vi "update_kineticslength_exp.vi"(1 "NewVal":dbl, 2 "cluster in":T1={"Kinetics"=[], "Spectrum"=[], "Experiments groups"=[], "GRAPH EXPERIMENTAL DATA"=[], "error out"={"status"=FALSE, "code"=0, "source"=""}, "group"=0, "exp selected"=0, "# exp"=0, "kinetics plot names"=[], "spectra plot names"=[], "FromToWave"={"FromWave"=0.0, "ToWave"=0.0}, "GRAPH EXPERIMENTAL DATA ref"=refnum, "timedelays"=[0.0, 0.0, 0.0, 0.0, 0.0, 0.0, 0.0, 0.06019061100911815, 0.0521779104562645, 0.045231877429679615, 0.03921051490799832, 0.033990728811568754, 0.029465811603150715, 0.025543260876973825, 0.02214288834180205, 0.01919518054014414, 0.016639877791965713, 0.014424742312398925, 0.012504490320209958, 0.010839866306230088, 0.009396840537117498, 0.008145913389103785, 0.00706151229029317, 0.006121468943269439, 0.005306566140927374, 0.004600144911132549, 0.003987763959109073, 0.0034569044455719407, 0.00299671406541447, 0.0025977851951783253, 0.0022519625739982996, 0.00195217658646366, 0.0016922987392150965, 0.0014670163768006634, 0.0012717240756200802, 0.0011024294957352762, 0.0009556717658856477, 0.0008284507332614981, 0.0007181656316962257, 0.0006225619144775864, 0.0005396851648867825, 0.00046784114226338394, 0.0004055611468220084, 0.0003515719951773376, 0.00030476999279031153, 0.00026419837125694315, 0.00022902772919263772, 0.0001985390768670671, 0.0001721091379728629, 0.00014919760805372974, 0.00012933610911736794], "wavelengths"=[0.0, 0.0, 0.0, 0.0, 0.0, 0.0, 0.0, 0.06019061100911815, 0.0521779104562645, 0.045231877429679615, 0.03921051490799832, 0.033990728811568754, 0.029465811603150715, 0.025543260876973825, 0.02214288834180205, 0.01919518054014414, 0.016639877791965713, 0.014424742312398925, 0.012504490320209958, 0.010839866306230088, 0.009396840537117498, 0.008145913389103785, 0.00706151229029317, 0.006121468943269439, 0.005306566140927374, 0.004600144911132549, 0.003987763959109073, 0.0034569044455719407, 0.00299671406541447, 0.0025977851951783253, 0.0022519625739982996, 0.00195217658646366, 0.0016922987392150965, 0.0014670163768006634, 0.0012717240756200802, 0.0011024294957352762, 0.0009556717658856477, 0.0008284507332614981, 0.0007181656316962257, 0.0006225619144775864, 0.0005396851648867825, 0.00046784114226338394, 0.0004055611468220084, 0.0003515719951773376, 0.00030476999279031153, 0.00026419837125694315, 0.00022902772919263772, 0.0001985390768670671, 0.0001721091379728629, 0.00014919760805372974, 0.00012933610911736794], "Experiment"=refnum, "Commentaires exp"=refnum, "FromToDelay"={"FromDelay"=0.0, "ToDelay"=0.0}, "cluster tasks DAQmx"={"Heater alaram task"="", "Laser shutter task"="", "Motor task"="", "Accelerator shutter task"="", "Relay key task"="", "Faraday cup task"=""}}) -> (0 "cluster out":T1={"Kinetics"=[], "Spectrum"=[], "Experiments groups"=[], "GRAPH EXPERIMENTAL DATA"=[], "error out"={"status"=FALSE, "code"=0, "source"=""}, "group"=0, "exp selected"=0, "# exp"=0, "kinetics plot names"=[], "spectra plot names"=[], "FromToWave"={"FromWave"=0.0, "ToWave"=0.0}, "GRAPH EXPERIMENTAL DATA ref"=refnum, "timedelays"=[0.0, 0.0, 0.0, 0.0, 0.0, 0.0, 0.0, 0.06019061100911815, 0.0521779104562645, 0.045231877429679615, 0.03921051490799832, 0.033990728811568754, 0.029465811603150715, 0.025543260876973825, 0.02214288834180205, 0.01919518054014414, 0.016639877791965713, 0.014424742312398925, 0.012504490320209958, 0.010839866306230088, 0.009396840537117498, 0.008145913389103785, 0.00706151229029317, 0.006121468943269439, 0.005306566140927374, 0.004600144911132549, 0.003987763959109073, 0.0034569044455719407, 0.00299671406541447, 0.0025977851951783253, 0.0022519625739982996, 0.00195217658646366, 0.0016922987392150965, 0.0014670163768006634, 0.0012717240756200802, 0.0011024294957352762, 0.0009556717658856477, 0.0008284507332614981, 0.0007181656316962257, 0.0006225619144775864, 0.0005396851648867825, 0.00046784114226338394, 0.0004055611468220084, 0.0003515719951773376, 0.00030476999279031153, 0.00026419837125694315, 0.00022902772919263772, 0.0001985390768670671, 0.0001721091379728629, 0.00014919760805372974, 0.00012933610911736794], "wavelengths"=[0.0, 0.0, 0.0, 0.0, 0.0, 0.0, 0.0, 0.06019061100911815, 0.0521779104562645, 0.045231877429679615, 0.03921051490799832, 0.033990728811568754, 0.029465811603150715, 0.025543260876973825, 0.02214288834180205, 0.01919518054014414, 0.016639877791965713, 0.014424742312398925, 0.012504490320209958, 0.010839866306230088, 0.009396840537117498, 0.008145913389103785, 0.00706151229029317, 0.006121468943269439, 0.005306566140927374, 0.004600144911132549, 0.003987763959109073, 0.0034569044455719407, 0.00299671406541447, 0.0025977851951783253, 0.0022519625739982996, 0.00195217658646366, 0.0016922987392150965, 0.0014670163768006634, 0.0012717240756200802, 0.0011024294957352762, 0.0009556717658856477, 0.0008284507332614981, 0.0007181656316962257, 0.0006225619144775864, 0.0005396851648867825, 0.00046784114226338394, 0.0004055611468220084, 0.0003515719951773376, 0.00030476999279031153, 0.00026419837125694315, 0.00022902772919263772, 0.0001985390768670671, 0.0001721091379728629, 0.00014919760805372974, 0.00012933610911736794], "Experiment"=refnum, "Commentaires exp"=refnum, "FromToDelay"={"FromDelay"=0.0, "ToDelay"=0.0}, "cluster tasks DAQmx"={"Heater alaram task"="", "Laser shutter task"="", "Motor task"="", "Accelerator shutter task"="", "Relay key task"="", "Faraday cup task"=""}})   [LabVIEW 2015]
uses:
  Classes/Experiment.lvclass
  Classes/Experiments_group.lvclass
  controls/control-cluster.ctl
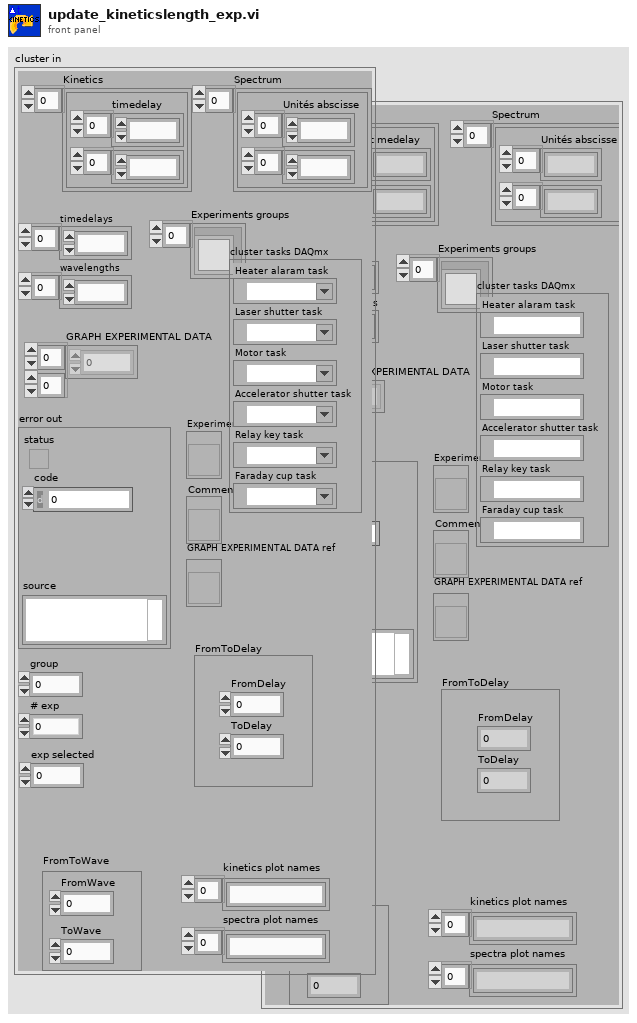
[diagram p1: front panel]
types:
  T1 = typedef "control-cluster.ctl" = cluster{"Kinetics":cluster{"timedelay":dbl[], dbl[]}[], "Spectrum":cluster{"Unités abscisse":dbl[], dbl[]}[], "Experiments groups":refnum<class "Experiments_group.lvclass">[], "GRAPH EXPERIMENTAL DATA":dbl[][], "error out":errorcluster, "group":i32, "exp selected":i32, "# exp":i32, "kinetics plot names":string[], "spectra plot names":string[], "FromToWave":cluster{"FromWave":dbl, "ToWave":dbl}, "GRAPH EXPERIMENTAL DATA ref":refnum<vi>, "timedelays":dbl[], "wavelengths":dbl[], "Experiment":refnum<vi>, "Commentaires exp":refnum<vi>, "FromToDelay":cluster{"FromDelay":dbl, "ToDelay":dbl}, "cluster tasks DAQmx":cluster{"Heater alaram task":refnum<k21>, "Laser shutter task":refnum<k21>, "Motor task":refnum<k21>, "Accelerator shutter task":refnum<k21>, "Relay key task":refnum<k21>, "Faraday cup task":refnum<k21>}}
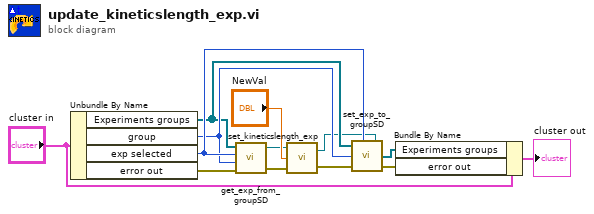
[diagram p0: block diagram]
diagram:
  n1 = Unbundle By Name("cluster in") -> ("Experiments groups"=w6:refnum<class "Experiments_group.lvclass">[], "group"=w7:i32, "exp selected"=w8:i32, "error out"=w1:errorcluster)
  n2 = call "get_exp_from_groupSD.vi"("error in (no error)"=w1, "group"=w7, "exp selected"=w8, "Experiments groups"=w6) -> ("error out"=w10:errorcluster, "Experiment out"=w4:refnum<class "Experiment.lvclass">)  [unwired: 1 out]
  n3 = call-dynamic "set_kineticslength_exp.vi"("error in (no error)"=w10, "KineticsLength, ps"="NewVal", "Experiment.lvclass in"=w4) -> ("error out"=w11:errorcluster, "Experiment.lvclass out"=w5:refnum<class "Experiment.lvclass">)
  n4 = call "set_exp_to_groupSD.vi"("Experiments groups"=w6, "exp selected"=w8, "group"=w7, "error in (no error)"=w11, "Experiment in"=w5) -> ("Experiments groups out"=w9:refnum<class "Experiments_group.lvclass">[], "error out"=w12:errorcluster)  [unwired: 1 in]
  n5 = Bundle By Name(cluster="cluster in", "Experiments groups"=w9, "error out"=w12) -> (→"cluster out":T1)
